vi "wa32 Flush Read.vi"(8 "error in":errorcluster, 11 "handle":i32) -> (0 "error out":errorcluster, 2 "read message":string, 3 "handle out":i32)   [LabVIEW 2020]
doc: "This VI will read all stuff from input."
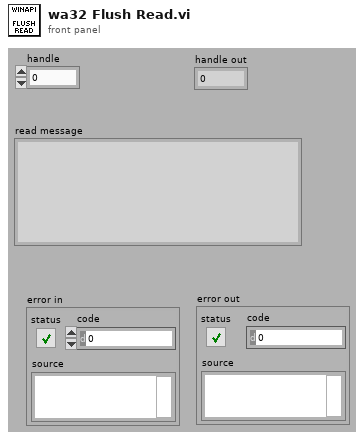
[diagram p1: front panel]
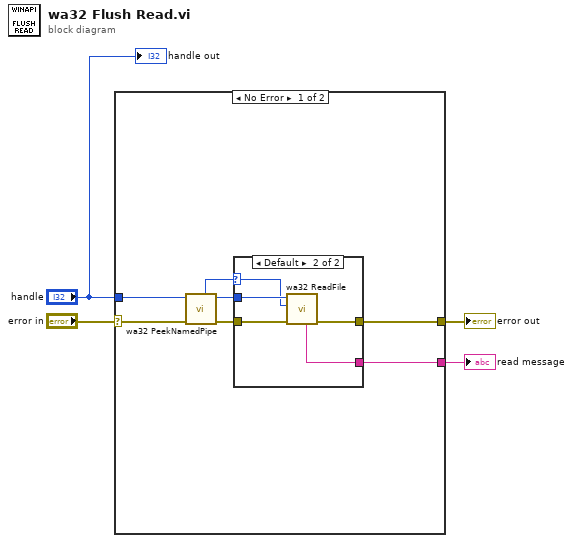
[diagram p0: block diagram]
diagram:
  n1 = case shown="No Error" "error in" {
    selector: "error in" -> [w11 w18]
    tunnel: "handle" -> [w10 _]
    tunnel: [w5 _] -> w3
    tunnel: [w6 w18] -> w2
    frame No Error {
      n2 = call "wa32 PeekNamedPipe.vi"("error in"=w11, "handle"=w10) -> ("error out"=w9:errorcluster, "handle out"=w8:i32, "available bytes"=w7:u32)  [unwired: 4 in, 3 out]
      n3 = case shown="Default" w7 {
        selector: w7 -> [_ w13]
        tunnel: w9 -> [w12 w17]
        tunnel: w8 -> [_ w16]
        tunnel: [w12 w15] -> w6
        tunnel: [_ w14] -> w5
        frame 0 {
        }
        frame Default {
          n4 = call "wa32 ReadFile.vi"("error in"=w17, "bytes to read (0)"=w13, "handle"=w16) -> ("error out"=w15:errorcluster, "read string"=w14:string)  [unwired: 4 in, 3 out]
        }
      }
    }
    frame Error {
    }
  }
  "read message" <- w3
  "error out" <- w2
  "handle out" <- "handle"
